vi "Actor Core.vi"(8 "error in":errorcluster, 11 "CS++SVMonitor in":refnum<class "CS++SVMonitor.lvclass">) -> (0 "error out":errorcluster, 3 "Actor out":refnum<class "Actor.lvclass">)   [LabVIEW 2013, in "CS++SVMonitor.lvlib" / "CS++SVMonitor.lvclass"]
doc: "(<B>Filename</B>: Actor Framework.lvlib:Actor.lvclass:Actor Core.vi)\n\nReceives messages to the actor, reacts to them, and initiates any error handling that may shut the actor down.\n\nDescendant classes may override this VI to append parallel tasks for the actor to complete while it handles messages. Overrides use the Call Parent Method node."
uses:
  CS++SVMonitor.lvclass
  <vilib>/ActorFramework/Actor/Actor.lvclass
  <vilib>/ActorFramework/Message Enqueuer/Message Enqueuer.lvclass
  CS++PVMonitor Messages/CS++PVUpdate Msg/CS++PVUpdate Msg.lvclass
  Classes/CS++ProcessVariables/ProcessVariable/PV.lvclass
  CS++PVMonitor/CS++PVMonitor.lvclass/CS++PVMonitor.ctl
  CS++BaseActor/CS++BaseActor.lvclass/CS++BaseActor.ctl
  CS++SVMonitor.lvclass/CS++SVMonitor.ctl
  CS++PVMonitor/CS++PVMonitor.lvclass
  Classes/CS++ProcessVariables/ProcessVariable/PV.lvclass/PV.ctl
  Classes/CS++ProcessVariables/ProcessVariable/Write PV URL.vi
  Classes/CS++ProcessVariables/ProcessVariable/Write Data.vi
  Classes/CS++ProcessVariables/ProcessVariable/Write Timestamp.vi
  Classes/CS++ProcessVariables/ProcessVariable/Write Error.vi
  Classes/CS++ProcessVariables/ProcessVariable/Write Quality.vi
  Classes/CS++ProcessVariables/ProcessVariable/Write status.vi
  CS++BaseActor/CS++BaseActor.lvclass
panel:
  out "Read Error":errorcluster
  out "Time Stamp Control":timestamp
  out "Data":variant
  out "PV URL":string
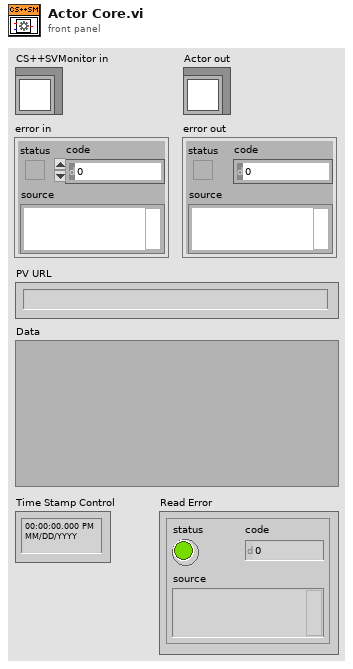
[diagram p1: front panel]
types:
  T1 = enum32{"Invalid", "Standard", "Closed", "Hidden", "Minimized", "Maximized"}
  T2 = cluster{"SV Refnums":refnum<k21>[], "PV Connections":cluster{"PV URL":string, "Observers":cluster{"Enqueuer":refnum<class "Message Enqueuer.lvclass">, "CS++PVUpdate Msg":refnum<class "CS++PVUpdate Msg.lvclass">}[]}[]}
  T3 = cluster{"Enqueuer":refnum<class "Message Enqueuer.lvclass">, "CS++PVUpdate Msg":refnum<class "CS++PVUpdate Msg.lvclass">}[]
  T4 = cluster{"PV URL":string, "Observers":cluster{"Enqueuer":refnum<class "Message Enqueuer.lvclass">, "CS++PVUpdate Msg":refnum<class "CS++PVUpdate Msg.lvclass">}[]}[]
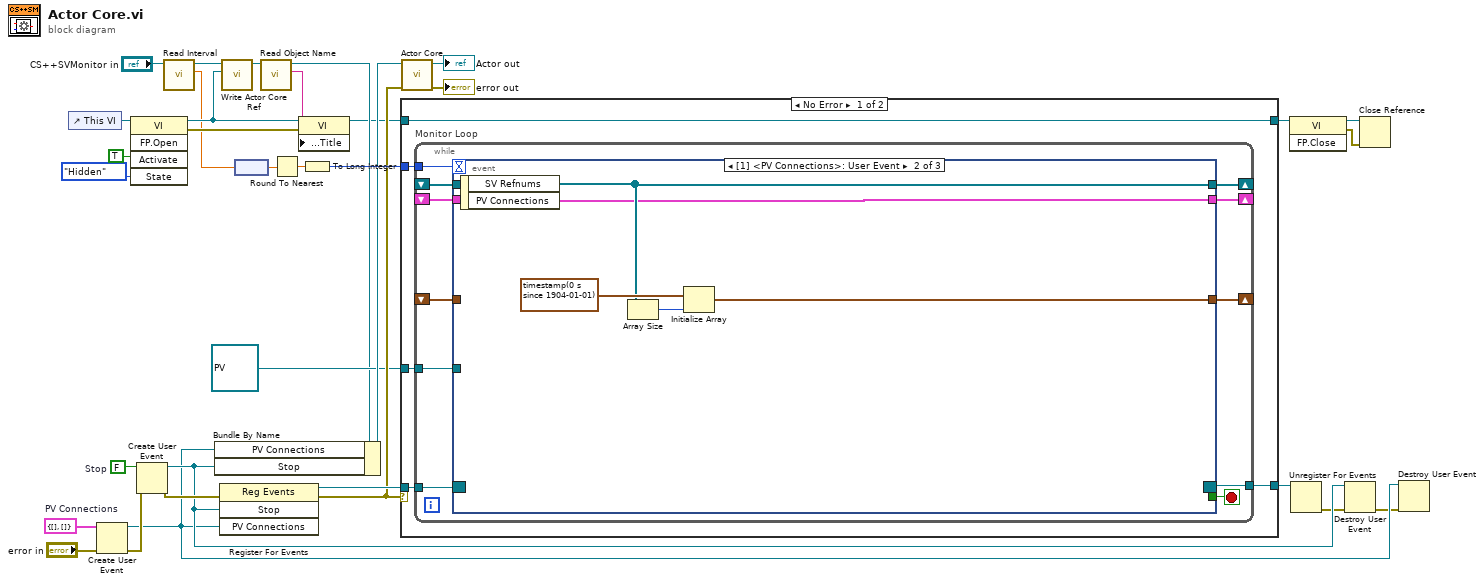
[diagram p0: block diagram]
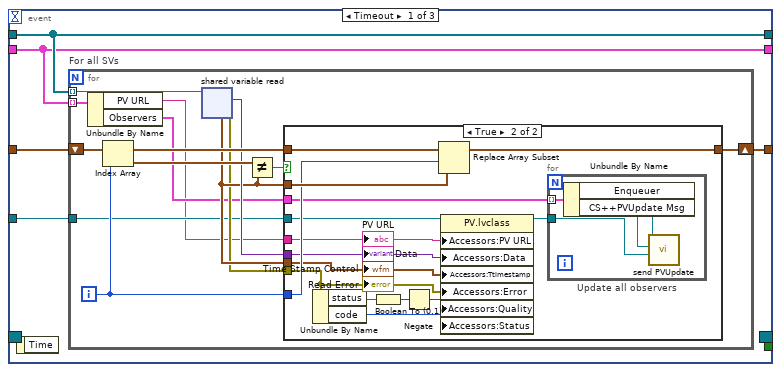
[diagram p2: hidden frame]
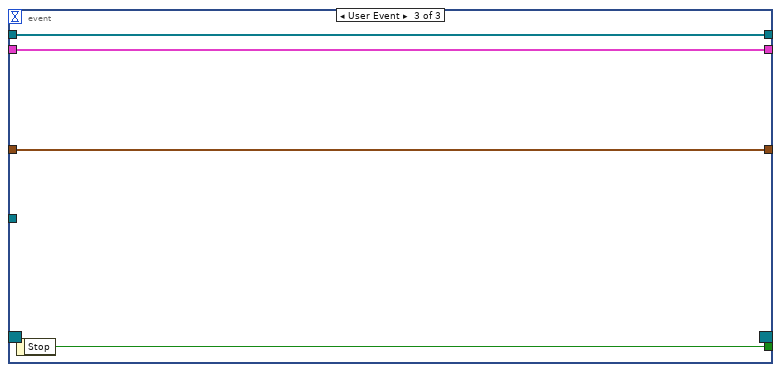
[diagram p4: hidden frame]
diagram:
  w17 = T2 {"SV Refnums"=[], "PV Connections"=[]}  # PV Connections
  w32 = FALSE  # Stop
  n1 = control-ref of="This VI"() -> (w15:refnum<vi>)
  n2 = Create User Event(user event datatype=w17, error in="error in") -> (user event=w24:refnum<user-event>, error out=w25:errorcluster)
  n3 = invoke class="VI" method="FP.Open"(reference=w15, "Activate"=TRUE ("Activate?"), "State"=T1."Hidden") -> (reference out=w9:refnum<vi>, error out=w11:errorcluster)  [unwired: 2 in, 3 out]
  n4 = Create User Event(user event datatype=w32, error in=w25) -> (user event=w26:refnum<user-event>, error out=w31:errorcluster)
  n5 = call "Read Interval.vi"("CS++PVMonitor in"="CS++SVMonitor in") -> ("Interval"=w1:dbl[unit], "CS++PVMonitor out"=w2:refnum<class "CS++SVMonitor.lvclass">)  [unwired: 8 in, 1 out]
  n6 = register-events(error in=w31, w26, w24) -> (reference out=w30:refnum<event-registration>, error out=w19:errorcluster)  [unwired: 1 in]
  n7 = call "Write Actor Core Ref.vi"("Actor Core Ref"=w9, "CS++BaseActor in"=w2) -> ("CS++BaseActor out"=w12:refnum<class "CS++SVMonitor.lvclass">)  [unwired: 8 in, 1 out]
  n8 = node(w1) -> (w29:dbl)
  n9 = call "Read Object Name.vi"("CS++BaseActor in"=w12) -> ("Object Name"=w10:string, "CS++BaseActor out"=w8:refnum<class "CS++SVMonitor.lvclass">)  [unwired: 8 in, 1 out]
  n10 = Bundle By Name(cluster=w8, "PV Connections"=w24, "Stop"=w26) -> (w20:refnum<class "CS++SVMonitor.lvclass">)
  n11 = Round To Nearest(number=w29) -> (nearest integer value=w28:dbl)
  n12 = property class="VI"(reference=w9, error in=w11, "Front Panel.Title"=w10) -> (reference out=w6:refnum<vi>)  [unwired: 1 out]
  n13 = To Long Integer(number=w28) -> (32bit integer=w27:i32)
  n14 = case shown="No Error" w19 {
    tunnel: w30 -> [w39 w99]
    tunnel: w27 -> [w38 _]
    tunnel: [w37 w99] -> w23
    tunnel: refnum<class "PV.lvclass"> refnum ("CS++ProcessVariables.lvlib:PV.lvclass") -> [w36 _]
    tunnel: [w35 w98] -> w7
    tunnel: w6 -> [w35 w98]
    frame No Error {
      n15 = while "Monitor Loop" {
        tunnel: w39 -> [w50]
        tunnel: w38 -> [w49]
        tunnel: [w47] -> w37
        shift-right: [w45] -> _
        shift-left: _ -> [w46]
        shift-right: [w43] -> _
        shift-left: _ -> [w44]
        shift-right: [w42] -> _
        shift-left: _ -> [w41]
        tunnel: w36 -> [w40]
        stop <- w48 stop-if-true
        n16 = event shown="[1] <PV Connections>: User Event" {
          selector: w50 -> [_ _ _]
          dyn-events: [_ _ _] -> w47
          timeout: w49 -> [_ _ _]
          tunnel: [_ _ w97] -> w48
          tunnel: w46 -> [w55 _ w96]
          tunnel: [w54 w90 w96] -> w45
          tunnel: w44 -> [w53 _ w95]
          tunnel: [w53 w91 w95] -> w43
          tunnel: [w51 w89 w94] -> w42
          tunnel: w41 -> [w51 _ w94]
          tunnel: w40 -> [w52 _ _]
          event Timeout {
            n17 = event-data() -> ()  [unwired: 1 in, 1 out]
            n18 = for "For all SVs" {
              shift-right: [w65] -> w54
              shift-left: w55 -> [w67]
              tunnel: w53 -> [w60] mode=indexing
              tunnel: w51 -> [w59] mode=indexing
              tunnel: w52 -> [w57]
              i -> [w66]
              n19 = Unbundle By Name(w59) -> ("PV URL"=w56:string, "Observers"=w58:T3)
              n20 = Index Array(array=w67, index=w66) -> (element=w68:timestamp)
              n21 = shared-variable-read(w60) -> (w61:errorcluster, w63:variant, w62:timestamp)  [unwired: 1 in, 1 out]
              n22 = Not Equal?(x=w68, y=w62) -> (x != y?=w64:bool)
              n23 = case shown="True" w64 {
                tunnel: w62 -> [_ w84]
                tunnel: w67 -> [w69 w83]
                tunnel: w66 -> [_ w82]
                tunnel: [w69 w81] -> w65
                tunnel: w63 -> [_ w77]
                tunnel: w62 -> [_ w76]
                tunnel: w61 -> [_ w75]
                tunnel: w58 -> [_ w80]
                tunnel: w57 -> [_ w79]
                tunnel: w56 -> [_ w70]
                frame False {
                }
                frame True {
                  n24 = Unbundle By Name(w75) -> ("status"=w74:bool, "code"=w71:i32)
                  n25 = Boolean To (0,1)(Boolean=w74) -> (0, 1=w73:i16)
                  n26 = Negate(x=w73) -> (-x=w72:i16)
                  n27 = Replace Array Subset(array=w83, new element=w84, index=w82) -> (w81:timestamp[])
                  n28 = property class="PV.lvclass"(reference=w79, "Accessors:PV URL"=w70, "Accessors:Data"=w77, "Accessors:Ttimestamp"=w76, "Accessors:Error"=w75, "Accessors:Quality"=w72, "Accessors:Status"=w71) -> (reference out=w78:refnum<class "PV.lvclass">)  [unwired: 1 in, 1 out]
                  n29 = for "Update all observers" {
                    tunnel: w80 -> [w88] mode=indexing
                    tunnel: w78 -> [w85]
                    n30 = Unbundle By Name(w88) -> ("Enqueuer"=w87:refnum<class "Message Enqueuer.lvclass">, "CS++PVUpdate Msg"=w86:refnum<class "CS++PVUpdate Msg.lvclass">)
                    n31 = call "send PVUpdate.vi"("PV"=w85, "CS++PVUpdate Msg in"=w86, "Message Enqueuer in"=w87) -> ()  [unwired: 7 in, 2 out]
                  }
                  "PV URL" <- w70
                  "Data" <- w77
                  "Time Stamp Control" <- w76
                  "Read Error" <- w75
                }
              }
            }
          }
          event User Event {
            n32 = event-data() -> ("SV Refnums"=w91:refnum<k21>[], "PV Connections"=w89:T4)  [unwired: 1 in]
            n33 = Array Size(array=w91) -> (size(s)=w93:i32)
            n34 = Initialize Array(timestamp(0 s since 1904-01-01) ("timestamp"), w93) -> (w90:timestamp[])
          }
          event User Event {
            n35 = event-data() -> ("Stop"=w97:bool)  [unwired: 1 in]
          }
        }
      }
    }
    frame Error {
    }
  }
  n36 = call-parent "Actor Core.vi"("error in"=w19, "CS++BaseActor in"=w20) -> ("error out"=→"error out":errorcluster, "Actor out"=→"Actor out":refnum<class "Actor.lvclass">)  [unwired: 8 in]
  n37 = invoke class="VI" method="FP.Close"(reference=w7) -> (reference out=w4:refnum<vi>, error out=w5:errorcluster)  [unwired: 2 in, 1 out]
  n38 = Unregister For Events(event registration refnum=w23) -> (error out=w22:errorcluster)  [unwired: 1 in]
  n39 = Destroy User Event(user event=w26, error in=w22) -> (error out=w21:errorcluster)
  n40 = Close Reference(reference=w4, error in (no error)=w5) -> ()  [unwired: 1 out]
  n41 = Destroy User Event(user event=w24, error in=w21) -> ()  [unwired: 1 out]
